vi "JoystickDeadZone.vi"() -> ()   [LabVIEW 2014]
panel:
  out "output variable":dbl
  in  "input variable":dbl
  in  "scale":dbl
  in  "dead zone":dbl
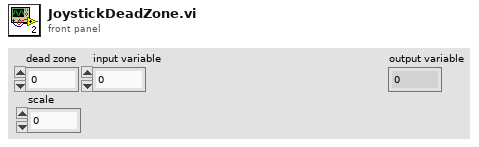
[diagram p1: front panel]
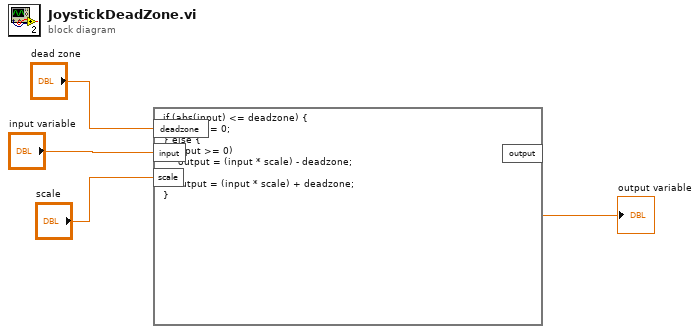
[diagram p0: block diagram]
diagram:
  n1 = formula code="if (abs(input) <= deadzone) {\n    output = 0;\n} else {\nif (input >= 0)\n     output = (input * scale) - deadzone;\nelse\n    output = (input * scale) + deadzone;\n}"("deadzone"="dead zone", "scale"="scale", "input"="input variable") -> ("output"=→"output variable":dbl)
